vi "pointinirons.vi"(9 "Absolute Wind Direction":dbl, 10 "Boat location":T1 {"North" format="%#_10f"; "East" format="%#_8f"}, 11 "PointA":T1 {"North" format="%#_10f"; "East" format="%#_8f"}) -> (3 "x <= y?":bool)   [LabVIEW 2013]
uses:
  Data/TypeDefs/UTM Location.ctl
panel:
  in  "Irons Range":dbl=45.0
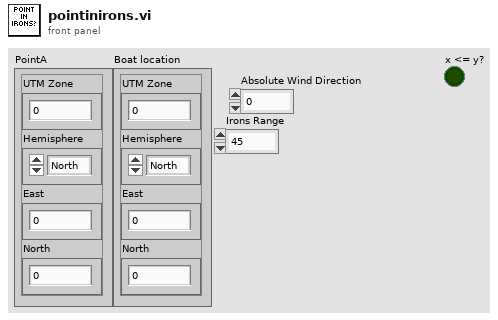
[diagram p1: front panel]
types:
  T1 = typedef "UTM Location.ctl" = cluster{"UTM Zone":dbl, "Hemisphere":enum16{"North", "South"}, "East":dbl, "North":dbl}
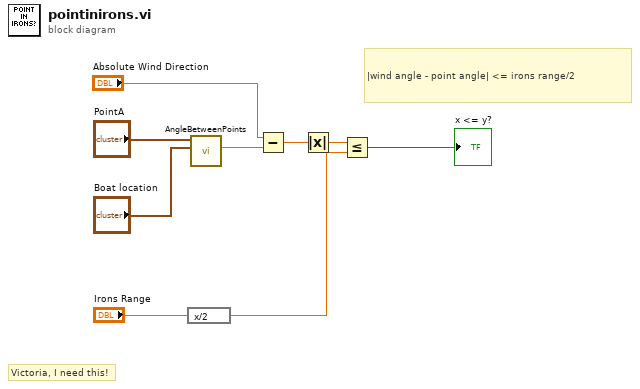
[diagram p0: block diagram]
diagram:
  # "|wind angle - point angle| <= irons range/2"
  # "Victoria, I need this!"
  n1 = expression code="x/2"("Irons Range") -> (w4:dbl)
  n2 = call "AngleBetweenPoints.vi"("Point 2"="Boat location", "Point 1"="PointA") -> ("Angle"=w6:dbl)  [unwired: 9 in]
  n3 = Subtract(x="Absolute Wind Direction", y=w6) -> (x-y=w2:dbl)
  n4 = Absolute Value(x=w2) -> (abs(x)=w1:dbl)
  n5 = Less Or Equal?(x=w1, y=w4) -> (x <= y?=→"x <= y?":bool)
